vi "Overlay Cross.vi"(5 "Color":u32(colorbox), 7 "error in (no error)":errorcluster, 8 "Overlay Group":string, 9 "point":cluster{"x":i16, "y":i16}, 10 "Image In":T1) -> (0 "error out":errorcluster, 3 "Image Out":T1)   [LabVIEW 2020, in "POLARIS Vision utility.lvlib"]
doc: "overlay a cross at specified point.\n\nauthor: Alexander Kessler, Helmholtz-Institut-Jena \nmaintainer: Alexander Kessler: alexander.kessler@uni-jena.de\n\n\n\nLicense Agreement for this software:\n\nCopyright (C)\nHelmholtz-Institut-Jena\nFröbelstieg 3\n07743 Jena\nGermany\n\nThis program is free software; you can redistribute it and/or modify it under the terms of the GNU General Public License as published by the Free Software Foundation; either version 2 of the license, or (at your option) any later version.\n\nThis program is distributed in the hope that it will be useful, but WITHOUT ANY WARRANTY; without even the implied warranty of MERCHANTABILITY or FITNESS FOR A PARTICULAR PURPOSE. See the GNU General License for more details (http://www.gnu.org)."
uses:
  POLARIS Vision utility.lvlib
  <vilib>/vision/Image Controls.llb/IMAQ Image.ctl
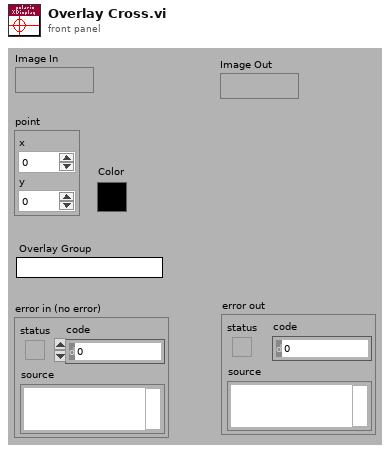
[diagram p1: front panel]
types:
  T1 = typedef "IMAQ Image.ctl" = refnum<image>
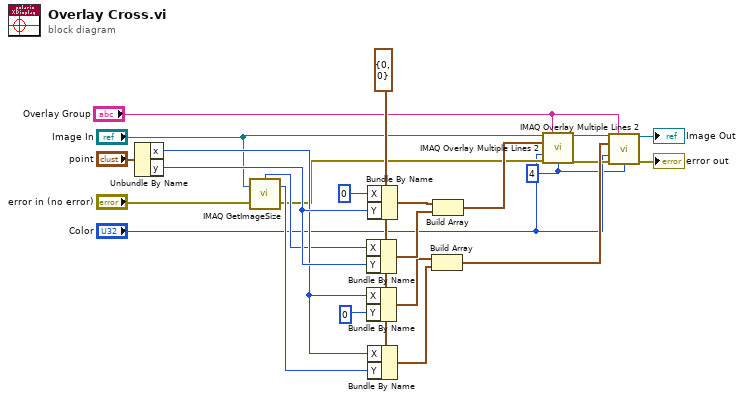
[diagram p0: block diagram]
diagram:
  w2 = u32 4 ("Width")
  w18 = cluster{"X":i32, "Y":i32} {"X"=0, "Y"=0} ("Start Point")
  n1 = Unbundle By Name("point") -> ("x"=w21:i16, "y"=w22:i16)
  n2 = call "IMAQ GetImageSize"("Image"="Image In", "error in (no error)"="error in (no error)") -> ("Y Resolution"=w19:i32, "X Resolution"=w20:i32, "error out"=w9:errorcluster)  [unwired: 2 in]
  n3 = Bundle By Name(cluster=w18, "X"=w20, "Y"=w22) -> (w14:cluster{"X":i32, "Y":i32})
  n4 = Bundle By Name(cluster=w18, "X"=w21, "Y"=0) -> (w13:cluster{"X":i32, "Y":i32})
  n5 = Bundle By Name(cluster=w18, "X"=0 ("Y"), "Y"=w22) -> (w15:cluster{"X":i32, "Y":i32})
  n6 = Bundle By Name(cluster=w18, "X"=w21, "Y"=w19) -> (w12:cluster{"X":i32, "Y":i32})
  n7 = Build Array(w13, w12) -> (w10:cluster{"X":i32, "Y":i32}[])
  n8 = Build Array(w15, w14) -> (w11:cluster{"X":i32, "Y":i32}[])
  n9 = call "IMAQ Overlay Multiple Lines 2"("Image"="Image In", "Group"="Overlay Group", "Line End Points"=w11, "Color"="Color", "error in (no error)"=w9, "Width"=w2) -> ("Image Out"=w6:T1, "error out"=w8:errorcluster)  [unwired: 8 in]
  n10 = call "IMAQ Overlay Multiple Lines 2"("Image"=w6, "Group"="Overlay Group", "Line End Points"=w10, "Color"="Color", "error in (no error)"=w8, "Width"=w2) -> ("Image Out"=→"Image Out":T1, "error out"=→"error out":errorcluster)  [unwired: 8 in]
